vi "MathUtil_Clamp_Int.vi"(9 "High":i32, 10 "Low":i32, 11 "Value":i32) -> (3 "Result":i32)   [LabVIEW 2019, in "Trajectory_Library.lvlib"]
doc: "Returns value clamped between low and high boundaries.\n \nInputs:\n - value -- Value to clamp.\n - low -- The lower boundary to which to clamp value.\n - high -- The higher boundary to which to clamp value.\n\nOutputs:\n - Result -- The clamped value."
uses:
  Trajectory_Library.lvlib
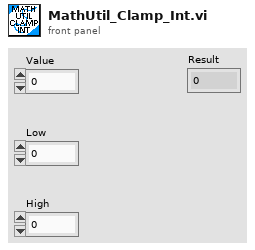
[diagram p1: front panel]
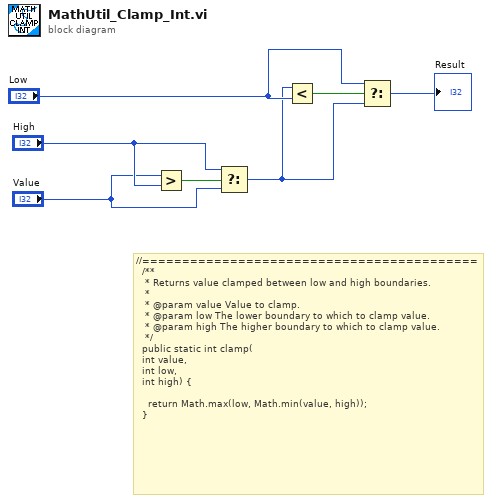
[diagram p0: block diagram]
diagram:
  # "//==========================================\n  /**\n   * Returns value clamped between low and high boundaries.\n   *\n   * @param value Value to clamp.\n   * @param low The lower boundary to which to clamp value.\n   * @param high The higher boundary to which to clamp value.\n   */\n  public static int clamp(\n\t\tint value, \n\t\tint low, \n\t\tint high) {\n\n    return Math.max(low, Math.min(value, high));\n  }"
  n1 = Greater?(x="Value", y="High") -> (0:w6:bool)
  n2 = Select(t="High", s=w6, f="Value") -> (s? t:f=w2:i32)
  n3 = Less?(x=w2, y="Low") -> (x < y?=w7:bool)
  n4 = Select(t="Low", s=w7, f=w2) -> (s? t:f=→"Result":i32)
